vi "Verify Analog Replay Settings.vi"(8 "error in (no error)":errorcluster, 10 "Analog Replay Data Options in":T1={"Input file"=path "", "Group"="", "Channel"="", "Reverse"=FALSE, "FPGA Memory Size"=enum."16,384", "Position reference"=enum."Crank angle", "Data selection method"=enum."Manual", "Offset"=0, "Samples"=0, "Missing teeth location"=0.0, "DataPlugin"=""}, 11 "Analog Replay Settings in":T5={"Name"="", "DAC bipolar range (V)"=0.0, "Voltage below min speed"=0.0, "Min speed (RPM)"=0.0, "Voltage at min speed"=0.0, "Max speed (RPM)"=0.0, "Voltage at max speed"=0.0, "Negate playback voltage values at negative engine speed"=TRUE, "Allow run-time override of voltage scaling"=FALSE}) -> (0 "error out":errorcluster, 2 "Analog Replay Data Options out":T1={"Input file"=path "", "Group"="", "Channel"="", "Reverse"=FALSE, "FPGA Memory Size"=enum."16,384", "Position reference"=enum."Crank angle", "Data selection method"=enum."Manual", "Offset"=0, "Samples"=0, "Missing teeth location"=0.0, "DataPlugin"=""}, 3 "Analog Replay Settings out":T5={"Name"="", "DAC bipolar range (V)"=0.0, "Voltage below min speed"=0.0, "Min speed (RPM)"=0.0, "Voltage at min speed"=0.0, "Max speed (RPM)"=0.0, "Voltage at max speed"=0.0, "Negate playback voltage values at negative engine speed"=TRUE, "Allow run-time override of voltage scaling"=FALSE})   [LabVIEW 2015, in "Engine Simulation Toolkit SysDef API.lvlib"]
uses:
  Engine Simulation Toolkit SysDef API.lvlib
  Analog Replay Settings.ctl
  Analog Replay Data Options.ctl
  System Explorer/FPGA Mem Size.ctl
  System Explorer/Position Reference.ctl
  System Explorer/Data Replay Data Selection Method.ctl
  System Explorer/Engine Simulation Toolkit System Explorer.lvlib
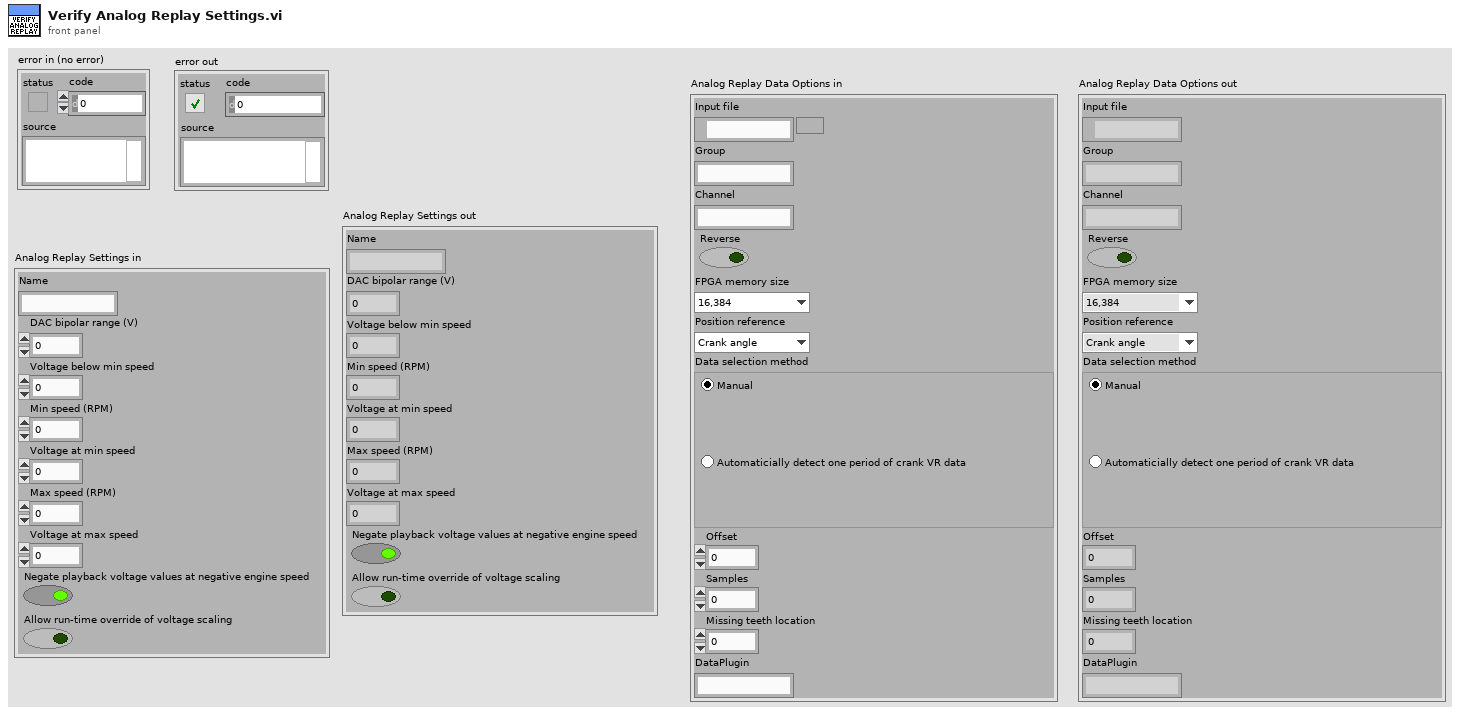
[diagram p1: front panel]
types:
  T1 = typedef "Engine Simulation Toolkit SysDef API.lvlib/Analog Replay Data Options.ctl" = cluster{"Input file":path, "Group":string, "Channel":string, "Reverse":bool, "FPGA Memory Size":T2, "Position reference":T3, "Data selection method":T4, "Offset":i32, "Samples":i32, "Missing teeth location":dbl, "DataPlugin":string}
  T2 = typedef "Engine Simulation Toolkit System Explorer.lvlib/FPGA Mem Size.ctl" = enum16{"65,536", "32,768", "16,384", "8,192", "4,096", "2,048", "1,024"}
  T3 = typedef "Engine Simulation Toolkit System Explorer.lvlib/Position Reference.ctl" = enum16{"Crank angle", "Cycle angle"}
  T4 = typedef "Engine Simulation Toolkit System Explorer.lvlib/Data Replay Data Selection Method.ctl" = enum32{"Manual", "AutoVRCrank"}
  T5 = typedef "Engine Simulation Toolkit SysDef API.lvlib/Analog Replay Settings.ctl" = cluster{"Name":string, "DAC bipolar range (V)":dbl, "Voltage below min speed":dbl, "Min speed (RPM)":dbl, "Voltage at min speed":dbl, "Max speed (RPM)":dbl, "Voltage at max speed":dbl, "Negate playback voltage values at negative engine speed":bool, "Allow run-time override of voltage scaling":bool}
  T6 = typedef "usiPluginInformation.ctl" = cluster{"name":string, "version":string, "type":string, "read-only?":bool, "extensions":string[]}
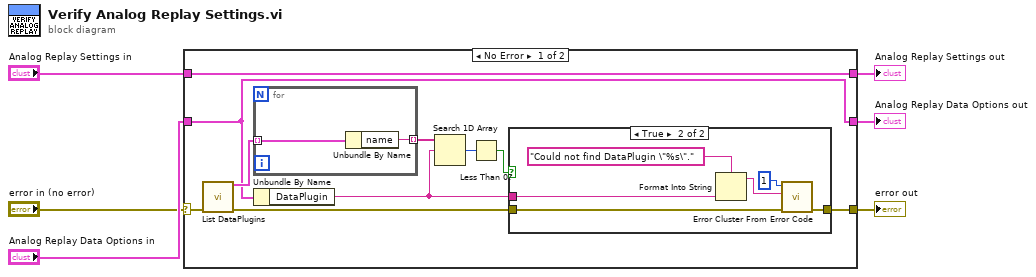
[diagram p0: block diagram]
diagram:
  n1 = case shown="No Error" "error in (no error)" {
    selector: "error in (no error)" -> [w9 w28]
    tunnel: "Analog Replay Data Options in" -> [w7 w26]
    tunnel: [w11 w28] -> w5
    tunnel: "Analog Replay Settings in" -> [w8 w27]
    tunnel: [w8 w27] -> w2
    tunnel: [w7 w26] -> w1
    frame No Error {
      n2 = call <vilib>:"List DataPlugins.vi"("error in (no error)"=w9) -> ("DataPlugin information"=w16:T6[], "error out"=w12:errorcluster)  [unwired: 13 in]
      n3 = for {
        tunnel: w16 -> [w25] mode=indexing
        tunnel: [w24] -> w15 mode=indexing
        n4 = Unbundle By Name(w25) -> ("name"=w24:string)
      }
      n5 = Unbundle By Name(w7) -> ("DataPlugin"=w10:string)
      n6 = Search 1D Array(1D array=w15, element=w10) -> (index of element=w14:i32)  [unwired: 1 in]
      n7 = Less Than 0?(x=w14) -> (x < 0?=w13:bool)
      n8 = case shown="True" w13 {
        tunnel: w12 -> [w17 w23]
        tunnel: [w17 w22] -> w11
        tunnel: w10 -> [_ w19]
        frame False {
        }
        frame True {
          n9 = Format Into String(format string="Could not find DataPlugin \"%s\"." ("error message (\"\")"), w19) -> (resulting string=w18:string)  [unwired: 2 in, 1 out]
          n10 = call <vilib>:"Error Cluster From Error Code.vi"("error in (no error)"=w23, "error message (\"\")"=w18, "error code (0)"=1) -> ("error out"=w22:errorcluster)  [unwired: 6 in]
        }
      }
    }
    frame Error {
    }
  }
  "error out" <- w5
  "Analog Replay Settings out" <- w2
  "Analog Replay Data Options out" <- w1
